vi "linFit.vi"(1 "b":sgl, 2 "m":sgl, 3 "x":sgl) -> (0 "xm+b":sgl)   [LabVIEW 2021]
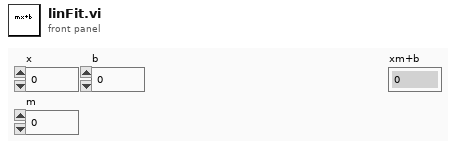
[diagram p1: front panel]
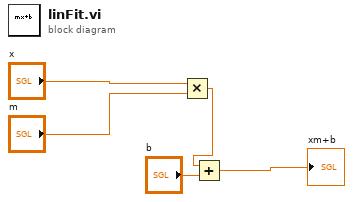
[diagram p0: block diagram]
diagram:
  n1 = Multiply(x="x", y="m") -> (x*y=w2:sgl)
  n2 = Add(x=w2, y="b") -> (x+y=→"xm+b":sgl)
